vi "SS2 Live_Decode FPGA Data.vi"(8 "Error In":errorcluster, 9 "Buffer Size (#8-bit Images)":i32, 10 "SS2 Live Internal Variables":T1={"okCFrontPanelDevices Refnum"=refnum, "Device Refnum"=refnum, "Display Image"=refnum, "# Live Images"=0, "relative s"=0.0, "# Image Sets"=0, "Message"="", "Current Image Set"=0, "# Datasets"=0, "Current Dataset"=0, "Live Mode"=FALSE, "Recording Mode"=FALSE, "Record Button"=refnum, "Live Button"=refnum, "SS2 Live Gate Data Q Name"="SS2 Live Gate Data Q", "Discard First Image"=FALSE, "Image Information"={"Save ROI Only"=FALSE, "Left"=0, "Top"=0, "Right"=0, "Bottom"=0, "Use Current ROI"=FALSE}, "Image Binning Options"={"Use Image Binning"=FALSE, "X Bin"=1, "Y Bin"=1}, "FPGA Serial Number"="", "PCB Version"=enum."PCB 1"} {"Image Binning Options"."Y Bin" min=1; "Image Binning Options"."X Bin" min=1}, 11 "FPGA Data Q":refnum<queue>) -> ()   [LabVIEW 2019]
uses:
  SS2 Live Internal Variables.ctl
  C:/UCLA Thinkpad Google Drive/LabVIEW 2019 SP1/builds/SS2 Live Distribution/Opal Kelly/C# Wrapper/libFrontPanel-csharp.dll
  Opal Kelly/C# Wrapper/libFrontPanel-csharp.dll
  <vilib>/vision/Image Controls.llb/IMAQ Image.ctl
  SS2 Live_Image ROI Information.ctl
  Phasor/Image Binning Options.ctl
  SS2 DAQ PCB Version.ctl
  8f499a87-0ce6-40db-98f3-8f764b7e409e.vi
  8d2e2152-5180-46c7-ad9e-0233ef769053.vi
  <vilib>/vision/NI_Vision_Development_Module.lvlib
  Notebook/Notebook.lvlib
  Rich Text Box/Rich Text Box.lvlib
panel:
  out "SS2 Live Internal Variables":T1={"okCFrontPanelDevices Refnum"=refnum, "Device Refnum"=refnum, "Display Image"=refnum, "# Live Images"=0, "relative s"=0.0, "# Image Sets"=0, "Message"="", "Current Image Set"=0, "# Datasets"=0, "Current Dataset"=0, "Live Mode"=FALSE, "Recording Mode"=FALSE, "Record Button"=refnum, "Live Button"=refnum, "SS2 Live Gate Data Q Name"="SS2 Live Gate Data Q", "Discard First Image"=FALSE, "Image Information"={"Save ROI Only"=FALSE, "Left"=0, "Top"=0, "Right"=0, "Bottom"=0, "Use Current ROI"=FALSE}, "Image Binning Options"={"Use Image Binning"=FALSE, "X Bin"=1, "Y Bin"=1}, "FPGA Serial Number"="", "PCB Version"=enum."PCB 1"} {"Image Binning Options"."Y Bin" min=1; "Image Binning Options"."X Bin" min=1}
  out "Activate Trigger Error Out":errorcluster
  out "8-bit Image Count":i32
  out "Error Out":errorcluster
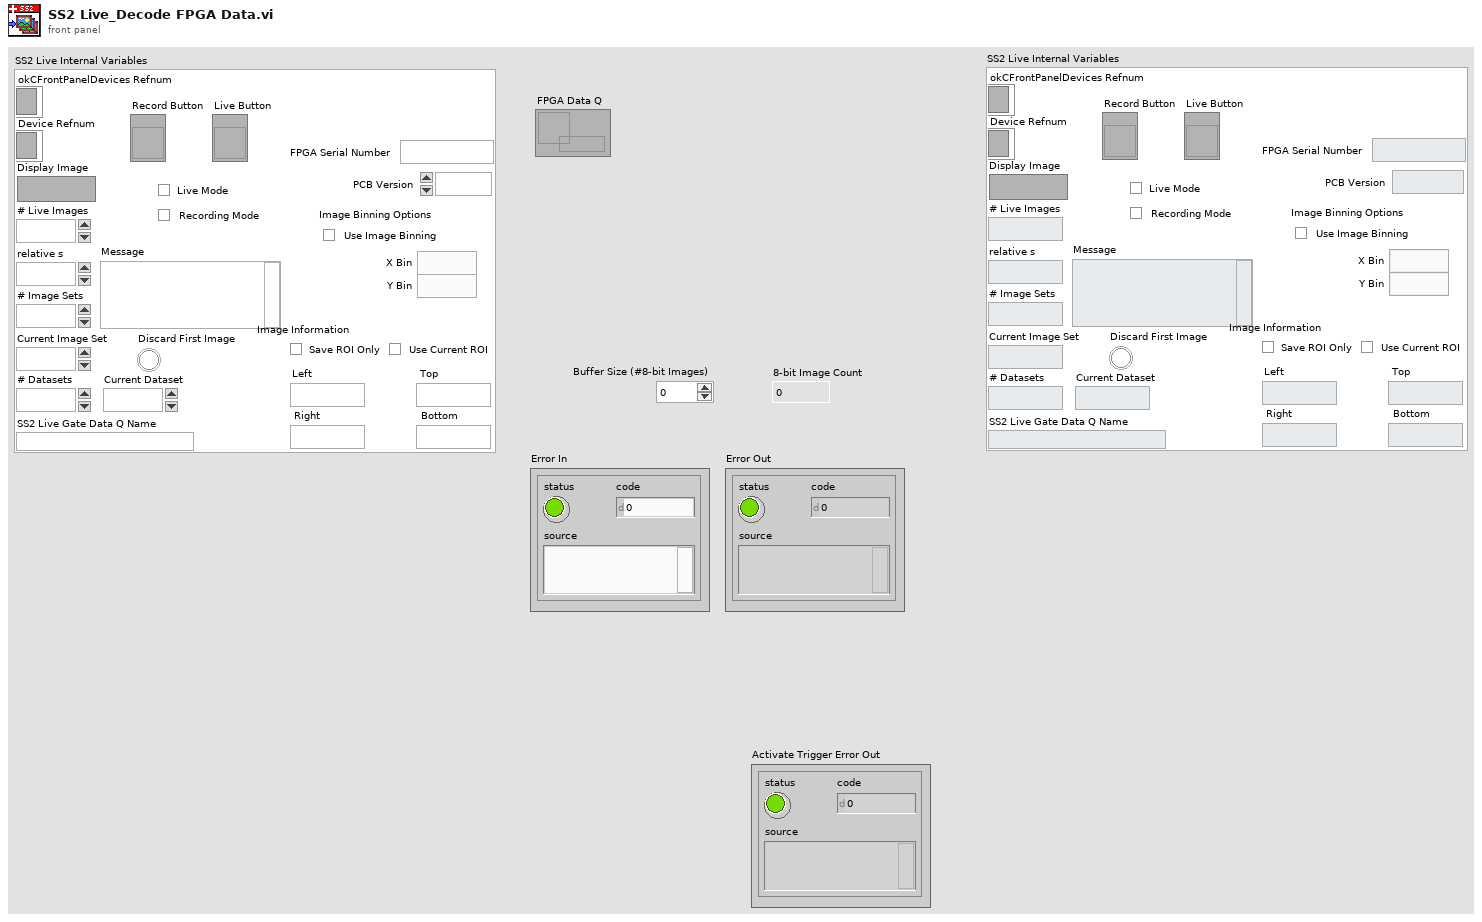
[diagram p1: front panel]
types:
  T1 = typedef "SS2 Live Internal Variables.ctl" = cluster{"okCFrontPanelDevices Refnum":refnum<k24>, "Device Refnum":refnum<k24>, "Display Image":T2, "# Live Images":i32, "relative s":dbl, "# Image Sets":i32, "Message":string, "Current Image Set":i32, "# Datasets":i32, "Current Dataset":i32, "Live Mode":bool, "Recording Mode":bool, "Record Button":refnum<vi>, "Live Button":refnum<vi>, "SS2 Live Gate Data Q Name":string, "Discard First Image":bool, "Image Information":T3, "Image Binning Options":T4, "FPGA Serial Number":string, "PCB Version":T5}
  T2 = typedef "IMAQ Image.ctl" = refnum<image>
  T3 = typedef "SS2 Live_Image ROI Information.ctl" = cluster{"Save ROI Only":bool, "Left":u16, "Top":u16, "Right":u16, "Bottom":u16, "Use Current ROI":bool}
  T4 = typedef "Image Binning Options.ctl" = cluster{"Use Image Binning":bool, "X Bin":i32, "Y Bin":i32}
  T5 = typedef "SS2 DAQ PCB Version.ctl" = enum16{"unknown", "PCB 1", "PCB 2"}
  T6 = typedef "Image Type" = u32
  T7 = typedef "Rich Text Box.lvlib/Text Formatting.ctl" = cluster{"Font":string, "Text Color":T8, "Text Background Color":T8, "Text Style":enum16{"Regular", "Bold", "Italic", "Underline", "Strikeout"}, "Font Size (Points)":dbl, "Text Alignment":i32}
  T8 = typedef "Rich Text Box.lvlib/Text Colors.ctl" = enum16{"Unchanged", "Black", "Blue", "Gray", "Green", "Red", "White"}
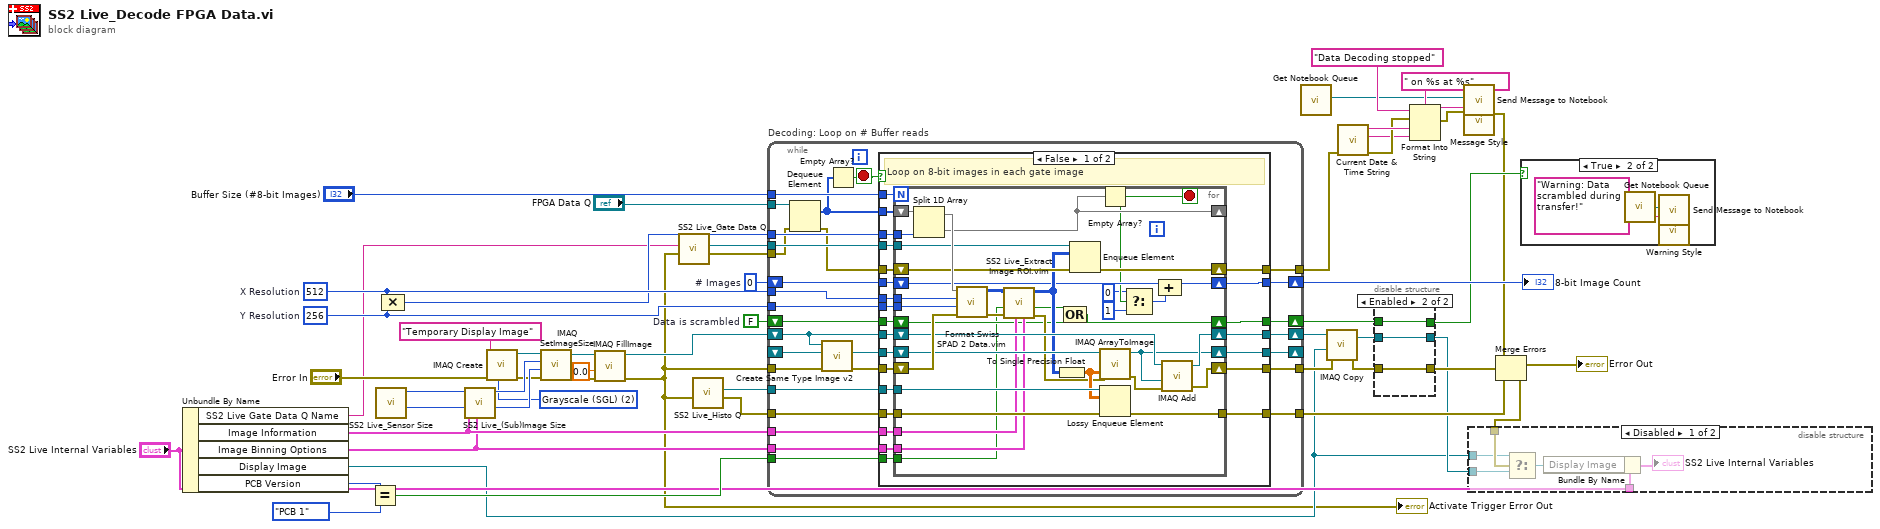
[diagram p0: block diagram]
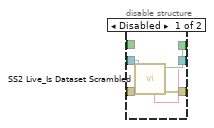
[diagram p3: hidden frame]
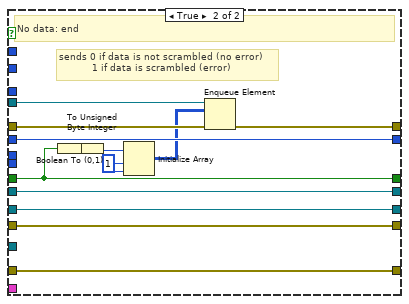
[diagram p5: hidden frame]
diagram:
  w24 = FALSE  # Data is scrambled
  w32 = T6 2 items=["Grayscale (U8)", "Grayscale (I16)", "Grayscale (SGL)", "Complex (CSG)", "RGB (U32)", "HSL (U32)", "RGB (U64)", "Grayscale (U16)"] ("Image Type")
  w48 = 0  # # Images
  w25 = 256  # Y Resolution
  w53 = 512  # X Resolution
  n1 = Unbundle By Name("SS2 Live Internal Variables") -> ("SS2 Live Gate Data Q Name"=w18:string, "Image Information"=w23:T3, "Image Binning Options"=w22:T4, "Display Image"=w14:T2, "PCB Version"=w21:T5)
  n2 = Equal?(x=w21, y=SS2_DAQ_PCB_Version."PCB 1" ("PCB Version")) -> (x = y?=w19:bool)
  n3 = call "SS2 Live_Sensor Size.vi"() -> ("Y size"=w33:i32, "X size"=w34:i32)  [unwired: 10 in]
  n4 = Compound Arithmetic op=MULTIPLY(w53, w25) -> (w30:i32)
  n5 = call "SS2 Live_(Sub)Image Size.vi"("Image Binning Options"=w22, "Image Information"=w23, "# Pixel Y in"=w33, "# Pixel X in"=w34) -> ("# Pixel Y out"=w46:i32, "# Pixel X out"=w47:i32)  [unwired: 6 in]
  n6 = call "IMAQ Create"("Image Name"="Temporary Display Image", "Image Type"=w32, "error in (no error)"="Error In") -> ("New Image"=w42:T2, "error out"=w44:errorcluster)  [unwired: 2 in]
  n7 = call "IMAQ SetImageSize"("error in (no error)"=w44, "Y Resolution"=w46, "X Resolution"=w47, "Image"=w42) -> ("error out"=w40:errorcluster, "Image Out"=w41:T2)  [unwired: 1 in]
  n8 = call "IMAQ FillImage"("error in (no error)"=w40, "Pixel Value (U8, U16, I16, Float)"=sgl 0.0, "Image"=w41) -> ("error out"=w13:errorcluster, "Image Out"=w39:T2)  [unwired: 7 in]
  "Activate Trigger Error Out" <- w13
  n9 = call "SS2 Live_Gate Data Q.vi"("error in (no error)"=w13, "SS2 Live Gate Data Q Name"=w18) -> ("error out"=w49:errorcluster, "SS2 Live Gate Data Q"=w54:refnum<queue>)  [unwired: 4 in]
  n10 = call "SS2 Live_Histo Q.vi"("error in (no error)"=w13) -> ("error out"=w51:errorcluster, "SS2 Live Histo Q"=w52:refnum<queue>)  [unwired: 5 in]
  n11 = while "Decoding: Loop on # Buffer reads" {
    tunnel: w25 -> [w83]
    tunnel: w53 -> [w82]
    tunnel: w13 -> [w75]
    tunnel: "Buffer Size (#8-bit Images)" -> [w81]
    tunnel: w30 -> [w80]
    shift-right: [w66] -> _
    shift-left: _ -> [w78]
    tunnel: [w79] -> w36
    tunnel: w54 -> [w73]
    tunnel: w49 -> [w64]
    tunnel: [w72] -> w5
    tunnel: w52 -> [w71]
    tunnel: w51 -> [w70]
    tunnel: [w69] -> w50
    shift-right: [w68] -> w37
    shift-left: w39 -> [w77]
    tunnel: "FPGA Data Q" -> [w65]
    shift-right: [w74] -> w45
    shift-left: w48 -> [w60]
    tunnel: w23 -> [w59]
    tunnel: w22 -> [w58]
    shift-right: [w57] -> w26
    shift-left: w24 -> [w56]
    tunnel: w19 -> [w55]
    stop <- w61 stop-if-true
    n12 = Dequeue Element(queue=w65, error in (no error)=w64) -> (element=w62:u8[], error out=w63:errorcluster)  [unwired: 1 in, 2 out]
    n13 = call "Create Same Type Image v2.vi"("error in (no error)"=w75, "Image Dst"=w78, "Image Src"=w77) -> ("error out"=w76:errorcluster, "Image Dst"=w67:T2)  [unwired: 6 in, 1 out]
    n14 = Empty Array?(array=w62) -> (empty?=w61:bool)
    n15 = case shown="False" w61 {
      tunnel: w83 -> [w107 _]
      tunnel: w82 -> [w106 _]
      tunnel: w81 -> [w105 _]
      tunnel: w80 -> [w104 _]
      tunnel: [w103 w153] -> w79
      tunnel: w77 -> [w102 w155]
      tunnel: w76 -> [w101 w153]
      tunnel: [w88 w156] -> w74
      tunnel: w73 -> [w100 w151]
      tunnel: [w99 w149] -> w72
      tunnel: w71 -> [w98 _]
      tunnel: w70 -> [w97 w152]
      tunnel: [w96 w152] -> w69
      tunnel: [w95 w155] -> w68
      tunnel: w67 -> [w94 w154]
      tunnel: [w93 w154] -> w66
      tunnel: w63 -> [w92 w150]
      tunnel: w62 -> [w91 _]
      tunnel: w60 -> [w89 w156]
      tunnel: w59 -> [w90 _]
      tunnel: w58 -> [w87 _]
      tunnel: [w85 w148] -> w57
      tunnel: w56 -> [w86 w148]
      tunnel: w55 -> [w84 _]
      frame False {
        # "Loop on 8-bit images in each gate image"
        n16 = for {
          N: w105 -> [_]
          tunnel: w107 -> [w143]
          tunnel: w106 -> [w142]
          shift-right: [w134] -> w103
          shift-left: w101 -> [w141]
          shift-right: [w133] -> _
          shift-left: w91 -> [w140]
          tunnel: w104 -> [w138]
          tunnel: w100 -> [w132]
          shift-right: [w130] -> w99
          shift-left: w92 -> [w131]
          tunnel: w98 -> [w129]
          tunnel: w97 -> [w128]
          tunnel: [w127] -> w96
          shift-right: [w125] -> w95
          shift-left: w102 -> [w136]
          shift-right: [w124] -> w93
          shift-left: w94 -> [w137]
          tunnel: w90 -> [w113]
          shift-right: [w118] -> w88
          shift-left: w89 -> [w119]
          tunnel: w87 -> [w112]
          shift-right: [w109] -> w85
          shift-left: w86 -> [w110]
          tunnel: w84 -> [w108]
          stop <- w117 stop-if-true
          n17 = Split 1D Array(array=w140, index=w138) -> (first subarray=w139:u8[], second subarray=w133:u8[])
          n18 = call "Format Swiss SPAD 2 Data.vim"("Error In"=w141, "Y Resolution"=w143, "X Resolution"=w142, "Flattened Image"=w139) -> ("Error Out"=w122:errorcluster, "Image out"=w123:u8[][])  [unwired: 6 in]
          n19 = call "SS2 Live_Extract Image ROI.vim"("Image Binning Options"=w112, "Image Information"=w113, "Error In"=w122, "Test for scrambling"=w108, "Image in"=w123) -> ("Error Out"=w121:errorcluster, "Data is scrambled"=w111:bool, "Image out"=w120:u8[][])  [unwired: 4 in]
          n20 = To Single Precision Float(number=w120) -> (single precision float=w126:sgl[][])
          n21 = Compound Arithmetic op=OR(w111, w110) -> (w109:bool)
          n22 = Enqueue Element(queue=w132, element=w120, error in (no error)=w131) -> (error out=w130:errorcluster)  [unwired: 1 in, 2 out]
          n23 = Empty Array?(array=w133) -> (empty?=w117:bool)
          n24 = call "IMAQ ArrayToImage"("Image Pixels (Float)"=w126, "error in (no error)"=w121, "Image"=w137) -> ("error out"=w135:errorcluster, "Image Out"=w124:T2)  [unwired: 7 in]
          n25 = Lossy Enqueue Element(queue=w129, element=w126, error in (no error)=w128) -> (error out=w127:errorcluster)  [unwired: 3 out]
          n26 = Select(t=0 ("value"), s=w117, f=1) -> (s? t:f=w116:i32)
          n27 = Compound Arithmetic op=ADD(w119, w116) -> (w118:i32)
          n28 = call "IMAQ Add"("Image Src A"=w136, "Image Src B"=w124, "error in (no error)"=w135) -> ("Image Dst Out"=w125:T2, "error out"=w134:errorcluster)  [unwired: 4 in]
        }
      }
      frame True {
        w145 = 1 ("dimension size")
        # "sends 0 if data is not scrambled (no error)\n           1 if data is scrambled (error)"
        # "No data: end"
        n29 = Boolean To (0,1)(Boolean=w148) -> (0, 1=w147:i16)
        n30 = To Unsigned Byte Integer(number=w147) -> (unsigned 8bit integer=w146:u8)
        n31 = Initialize Array(w146, w145, w145) -> (w144:u8[][])
        n32 = Enqueue Element(queue=w151, element=w144, error in (no error)=w150) -> (error out=w149:errorcluster)  [unwired: 1 in, 2 out]
      }
    }
  }
  "8-bit Image Count" <- w45
  n33 = call "Get Notebook Queue.vi"() -> ("Notebook Queue"=w6:refnum<queue>)  [unwired: 9 in]
  n34 = call "IMAQ Copy"("error in (no error)"=w36, "Image Dst"=w14, "Image Src"=w37) -> ("error out"=w29:errorcluster, "Image Dst Out"=w15:T2)  [unwired: 3 in]
  n35 = call "Current Date & Time String.vi"("Error In"=w5) -> ("Error Out"=w4:errorcluster, "time string"=w1:string, "date string"=w9:string)  [unwired: 8 in]
  n36 = disable-structure shown="Enabled" {
    disable-tunnel: w29 -> [w161 w163]
    disable-tunnel: [w160 w163] -> w28
    disable-tunnel: w15 -> [w159 w164]
    disable-tunnel: [w158 w162] -> w27
    disable-tunnel: [w157 w164] -> _
    disable-tunnel: w26 -> [_ w162]
    frame Disabled {
      n37 = call "SS2 Live_Is Dataset Scrambled.vi"("Error In"=w161, "Refnum in"=w159) -> ("Error Out"=w160:errorcluster, "SS2 image is scrambled"=w158:bool, "Warning"=w157:string)  [unwired: 4 in, 3 out]
    }
    frame Enabled {
    }
  }
  n38 = Format Into String(format string=" on %s at %s", initial string="Data Decoding stopped" ("Message"), error in=w4, w9, w1) -> (resulting string=w8:string, error out=w3:errorcluster)
  n39 = call "Message Style.vi"() -> ("Message Formatting"=w7:T7)
  n40 = call "Send Message to Notebook.vi"("Notebook Queue"=w6, "Message"=w8, "Error In"=w3, "Text Formatting"=w7) -> ("Error Out"=w2:errorcluster)  [unwired: 15 in]
  n41 = Merge Errors(w2, w28, w50) -> (w16:errorcluster)
  "Error Out" <- w16
  n42 = disable-structure shown="Disabled" {
    disable-tunnel: "SS2 Live Internal Variables" -> [w170 _]
    disable-tunnel: w16 -> [w168 _]
    disable-tunnel: w15 -> [w167 _]
    disable-tunnel: w14 -> [w166 _]
    frame Disabled {
      n43 = Select(t=w166, s=w168, f=w167) -> (s? t:f=w165:T2)
      n44 = Bundle By Name(cluster=w170, "Display Image"=w165) -> (→"SS2 Live Internal Variables":T1)
    }
    frame Enabled {
    }
  }
  n45 = case shown="True" w27 {
    frame False {
    }
    frame True {
      n46 = call "Get Notebook Queue.vi"() -> ("Notebook Queue"=w171:refnum<queue>)  [unwired: 9 in]
      n47 = call "Warning Style.vi"() -> ("Error Formatting"=w173:T7)
      n48 = call "Send Message to Notebook.vi"("Notebook Queue"=w171, "Message"="Warning: Data scrambled during transfer!" ("format string"), "Text Formatting"=w173) -> ()  [unwired: 16 in, 1 out]
    }
  }
